vi "get status.vi"(8 "error in (no error)":errorcluster, 10 "status":T1, 11 "id":i32) -> (0 "error out":errorcluster, 2 "status out":T1, 3 "function return":i32)   [LabVIEW 2017, in "libximc.lvlib"]
doc: "result_t XIMC_API get_status (device_t id, status_t* status);"
uses:
  libximc.lvlib
  libximc.dll
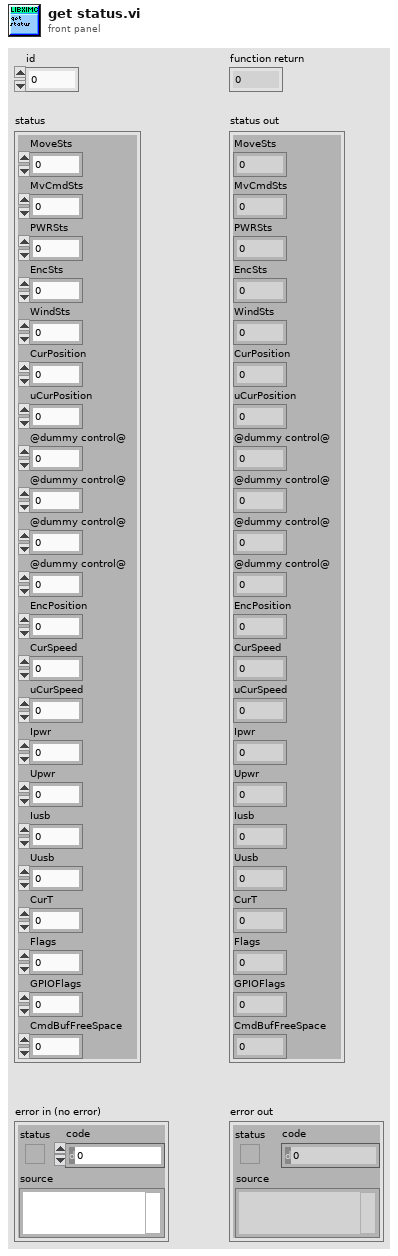
[diagram p1: front panel]
types:
  T1 = cluster{"MoveSts":u32, "MvCmdSts":u32, "PWRSts":u32, "EncSts":u32, "WindSts":u32, "CurPosition":i32, "uCurPosition":i32, "@dummy control@":i8, "@dummy control@":i8, "@dummy control@":i8, "@dummy control@":i8, "EncPosition":i64, "CurSpeed":i32, "uCurSpeed":i32, "Ipwr":i32, "Upwr":i32, "Iusb":i32, "Uusb":i32, "CurT":i32, "Flags":u32, "GPIOFlags":u32, "CmdBufFreeSpace":u32}
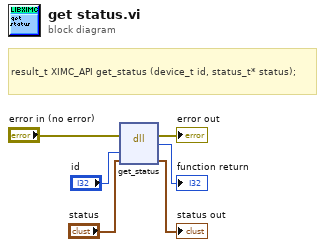
[diagram p0: block diagram]
diagram:
  # "result_t XIMC_API get_status (device_t id, status_t* status);"
  n1 = dll-call lib="C:/Users/francesco/dev/pump-probe/Stage/ximcLVx64/libximc.*" fn="get_status"(error in="error in (no error)", "id"="id", "status"="status") -> (error out=→"error out":errorcluster, →"function return":i32, "status"=→"status out":T1)  [unwired: 3 in, 1 out]
